vi "Parse Error Code from VI Name.vi"(11 "Call Chain":string[](array[string])) -> (3 "Error Code":i32)   [LabVIEW 2025, in "Error Helpers.lvlib"]
uses:
  Error Helpers.lvlib
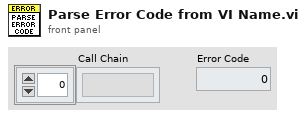
[diagram p1: front panel]
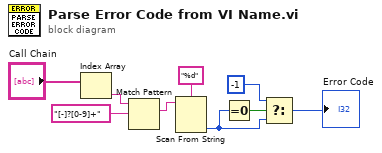
[diagram p0: block diagram]
diagram:
  n1 = Index Array(array="Call Chain") -> (element=w7:string)  [unwired: 1 in]
  n2 = Match Pattern(string=w7, regular expression="[-]?[0-9]+") -> (match substring=w8:string)  [unwired: 1 in, 3 out]
  n3 = Scan From String(format string="%d", input string=w8) -> (output 1=w2:i32)  [unwired: 3 in, 3 out]
  n4 = Equal To 0?(x=w2) -> (x = 0?=w3:bool)
  n5 = Select(t=-1, s=w3, f=w2) -> (s? t:f=→"Error Code":i32)
